vi "browseVariantArray.vi"(4 "Array of Variants":variant[](array[variant]), 6 "error in":errorcluster, 7 "ParentTag":string, 9 "VariantProbe.lvclass in":refnum<class "VariantTree__VP.lvclass">) -> (0 "error out":errorcluster, 3 "VariantProbe.lvclass out":refnum<class "VariantTree__VP.lvclass">)   [LabVIEW 2011, in "VariantTree__VP.lvclass"]
uses:
  VariantTree__VP.lvclass
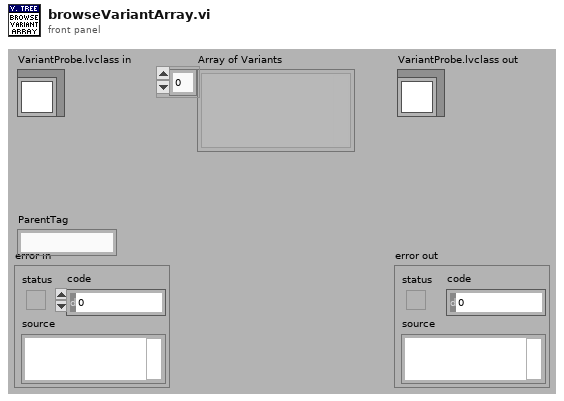
[diagram p1: front panel]
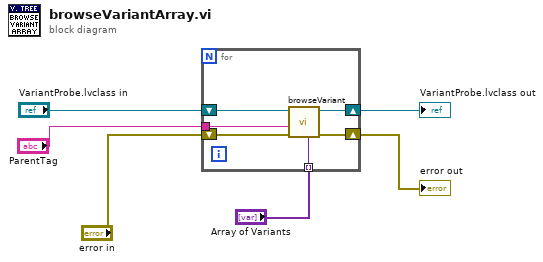
[diagram p0: block diagram]
diagram:
  n1 = for {
    tunnel: "ParentTag" -> [w8]
    shift-right: [w12] -> w4
    shift-left: "VariantProbe.lvclass in" -> [w9]
    tunnel: "Array of Variants" -> [w11] mode=indexing
    shift-right: [w10] -> w5
    shift-left: "error in" -> [w7]
    n2 = call-dynamic "browseVariant.vi"("Variant"=w11, "error in (no error)"=w7, "ParentTag"=w8, "VariantProbe.lvclass in"=w9) -> ("error out"=w10:errorcluster, "VariantProbe.lvclass out"=w12:refnum<class "VariantTree__VP.lvclass">)  [unwired: 4 in]
  }
  "error out" <- w5
  "VariantProbe.lvclass out" <- w4
